vi "az_to_rad_straight.vi"(1 "az quantity":u8, 2 "az":u8) -> (0 "rad":dbl)   [LabVIEW 2015]
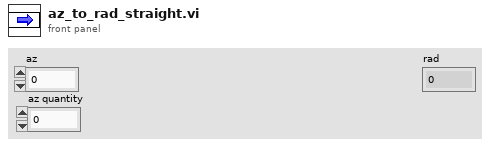
[diagram p1: front panel]
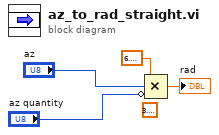
[diagram p0: block diagram]
diagram:
  (unwired) 3.141592653589793
  n1 = Compound Arithmetic op=MULTIPLY(6.283185307179586, "az", invert "az quantity") -> (→"rad":dbl)
